vi "Add_Projection_Layer.vi"(4 "seed":i32=42, 6 "Proj_Dim":i32=256, 8 "error in (no error)":errorcluster, 11 "NN in":T1 {"LR_Update_Policy"."WarmUp_Ratio" min=1; "LR_Update_Policy"."WarmUp_Iter" min=1; "LR_Update_Policy"."LR0" format="%.7f"}) -> (0 "error out":errorcluster, 3 "NN out":T1 {"LR_Update_Policy"."WarmUp_Ratio" min=1; "LR_Update_Policy"."WarmUp_Iter" min=1; "LR_Update_Policy"."LR0" format="%.7f"})   [LabVIEW 2020]
uses:
  <vilib>/Ngene/Deep Learning Toolkit/Toolkit/NN_Network/Controls/NN.ctl
  <vilib>/Ngene/Deep Learning Toolkit/Toolkit/NN_Layers/Controls/NN_Layer_ref.ctl
  <vilib>/Ngene/Deep Learning Toolkit/Toolkit/NN_Layers/Controls/NN_Layer.ctl
  <vilib>/Ngene/Deep Learning Toolkit/Toolkit/NN_Layers/Controls/NN_Layer_Type.ctl
  <vilib>/Ngene/Deep Learning Toolkit/Toolkit/NN_Data/API/NN_Dims(C,H,W).ctl
  <vilib>/Ngene/Deep Learning Toolkit/Toolkit/NN_Layers/Controls/NN_Layer_Metrics.ctl
  <vilib>/Ngene/Deep Learning Toolkit/Toolkit/NN_Network/Controls/NN_Device.ctl
  <vilib>/Ngene/Deep Learning Toolkit/Toolkit/NNg/cuda/Controls/nng_cuda_handles.ctl
  <vilib>/Ngene/Deep Learning Toolkit/Toolkit/NN_Layers/Controls/NN_Layer_Dimty.ctl
  <vilib>/Ngene/Deep Learning Toolkit/Toolkit/NN_Layers/Controls/NN_Layer_RF_State.ctl
  <vilib>/Ngene/Deep Learning Toolkit/Toolkit/NN_Data/API/NN_Dims(V,H).ctl
  <vilib>/Ngene/Deep Learning Toolkit/Toolkit/NN_Network/Controls/NN_In_Out_Dim-ty.ctl
  <vilib>/Ngene/Deep Learning Toolkit/Toolkit/NN_Train/Controls/NN_Train_Params.ctl
  <vilib>/Ngene/Deep Learning Toolkit/Toolkit/NN_Train/Controls/NN_Train_Optimizer.ctl
  <vilib>/Ngene/Deep Learning Toolkit/Toolkit/NN_Train/Controls/NN_Train_Data_Sampling.ctl
  <vilib>/Ngene/Deep Learning Toolkit/Toolkit/NN_Train/Controls/NN_LR_Policy_Cfg.ctl
  <vilib>/Ngene/Deep Learning Toolkit/Toolkit/NN_Train/Controls/NN_LR_Policy_Type.ctl
  <vilib>/Ngene/Deep Learning Toolkit/Toolkit/NN_Train/Controls/NN_Train_Session_Data.ctl
  <vilib>/Ngene/Deep Learning Toolkit/Toolkit/NN_Data/Controls/NN_Ground_truth.ctl
  <vilib>/Ngene/Deep Learning Toolkit/Toolkit/NN_Train/Controls/NN_Loss_Type.ctl
  <vilib>/Ngene/Deep Learning Toolkit/Toolkit/NNg/Network/WS/Controls/NNG_WS.ctl
  <vilib>/Ngene/Deep Learning Toolkit/Toolkit/NNg/Network/WS/Controls/NNg_WS_Mem_DVR.ctl
  <vilib>/Ngene/Deep Learning Toolkit/Toolkit/NNg/cuda/Controls/cuda_Mem_desc.ctl
  <vilib>/Ngene/Deep Learning Toolkit/Toolkit/NN_Layers/Layers/Conv2D/Controls/NN_Layer_Config(Conv2D).ctl
  <vilib>/Ngene/Deep Learning Toolkit/Toolkit/NN_Layers/Layers/Conv2D/Controls/NN_Layer_Params(Conv2D).ctl
  <vilib>/Ngene/Deep Learning Toolkit/Toolkit/NN_Layers/Layers/Conv2D/Controls/NN_Conv2D_Padding_Type.ctl
  <vilib>/Ngene/Deep Learning Toolkit/Toolkit/NN_Layers/Layers/BatchNorm/Controls/NN_BN_Params.ctl
  <vilib>/Ngene/Deep Learning Toolkit/Toolkit/NN_Activations/Controls/NN_Activation_Type.ctl
  <vilib>/Ngene/Deep Learning Toolkit/Toolkit/NN_Layers/Controls/NN_Layer_Init_Params.ctl
  <vilib>/Ngene/Deep Learning Toolkit/Toolkit/NN_Layers/Controls/NN_Layer_Weight_Init_Type.ctl
  <vilib>/Ngene/Deep Learning Toolkit/Toolkit/NN_Layers/Layers/Conv2D/NN_Layer_Create(Conv2D).vi
  <vilib>/Ngene/Deep Learning Toolkit/Toolkit/NN_Layers/subVIs/Get_Weights/NN_Get_Weights(Conv2D).vi
  <vilib>/Ngene/Deep Learning Toolkit/Toolkit/NN_Data/subVIs/Get_Data_Vals/2D/NN_Data_Get_ValByRef(2D_SGL).vi
  <vilib>/Ngene/Deep Learning Toolkit/Toolkit/NN_Data/subVIs/Set_Data_Vals/2D/NN_Data_Set_ValByRef(2D_SGL).vi
  <vilib>/Ngene/Deep Learning Toolkit/Toolkit/Deep_Learning_Toolkit_by_Ngene.lvlib
  <vilib>/Analysis/NI_AALBase.lvlib
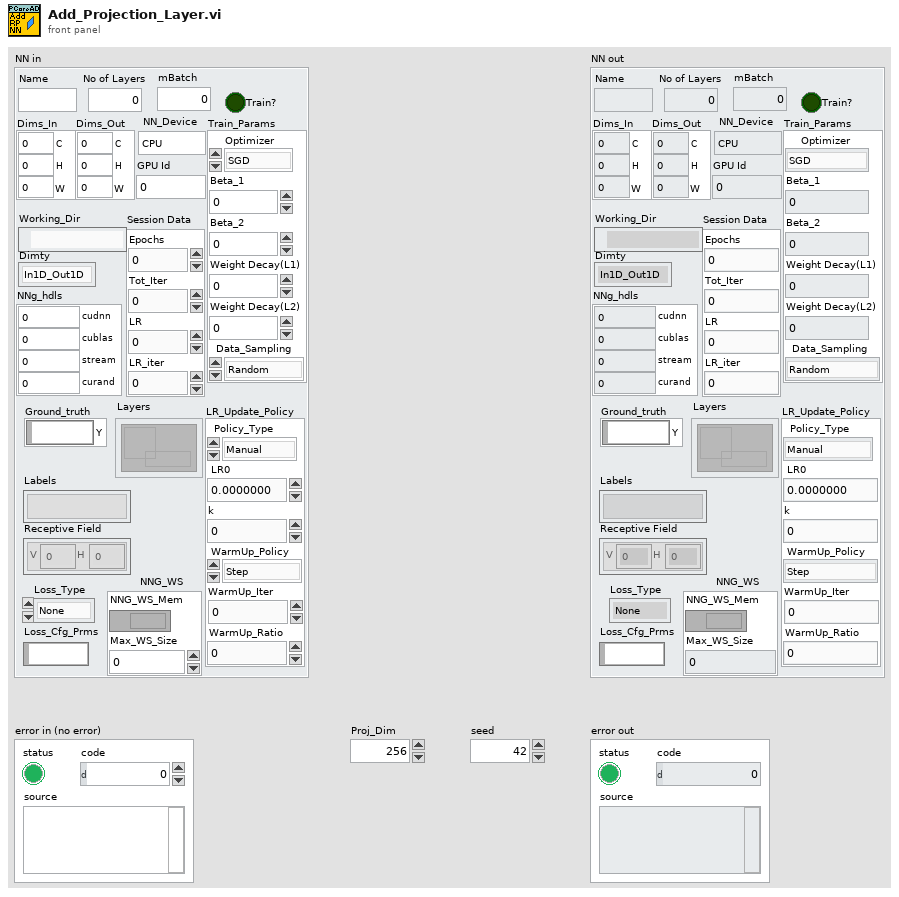
[diagram p1: front panel]
types:
  T1 = typedef "Deep_Learning_Toolkit_by_Ngene.lvlib/NN.ctl" = cluster{"Name":string, "No of Layers":i32, "mBatch":i32, "Layers":T2[], "Dimty":T3, "Dims_In":T4, "Dims_Out":T4, "Working_Dir":path, "Train?":bool, "Train_Params":T5, "LR_Update_Policy":T8, "Session Data":T10, "Ground_truth":T11, "NNg_hdls":T12, "NN_Device":T13, "GPU Id":i32, "Labels":string[], "Receptive Field":T14[], "Loss_Type":T15, "Loss_Cfg_Prms":variant, "NNG_WS":T16}
  T2 = typedef "Deep_Learning_Toolkit_by_Ngene.lvlib/NN_Layer_ref.ctl" = refnum<data-value>
  T3 = typedef "Deep_Learning_Toolkit_by_Ngene.lvlib/NN_In_Out_Dim-ty.ctl" = enum8{"In1D_Out1D", "In3D_Out1D", "In3D_Out3D", "In3D_OutBBox"}
  T4 = typedef "Deep_Learning_Toolkit_by_Ngene.lvlib/NN_Dims(C,H,W).ctl" = cluster{"C":i32, "H":i32, "W":i32}
  T5 = typedef "Deep_Learning_Toolkit_by_Ngene.lvlib/NN_Train_Params.ctl" = cluster{"Optimizer":T6, "Beta_1":sgl, "Beta_2":sgl, "Weight Decay(L1)":sgl, "Weight Decay(L2)":sgl, "Data_Sampling":T7}
  T6 = typedef "Deep_Learning_Toolkit_by_Ngene.lvlib/NN_Train_Optimizer.ctl" = enum16{"SGD", "Adam", "Adagrad", "Adadelta", "RMSProp", "Nesterov"}
  T7 = typedef "Deep_Learning_Toolkit_by_Ngene.lvlib/NN_Train_Data_Sampling.ctl" = enum16{"Random", "Sequential"}
  T8 = typedef "Deep_Learning_Toolkit_by_Ngene.lvlib/NN_LR_Policy_Cfg.ctl" = cluster{"Policy_Type":T9, "LR0":dbl, "k":sgl, "WarmUp_Policy":enum16{"Step", "Ramp"}, "WarmUp_Iter":i32, "WarmUp_Ratio":sgl}
  T9 = typedef "Deep_Learning_Toolkit_by_Ngene.lvlib/NN_LR_Policy_Type.ctl" = enum16{"Manual", "Step", "Exp", "1/t"}
  T10 = typedef "Deep_Learning_Toolkit_by_Ngene.lvlib/NN_Train_Session_Data.ctl" = cluster{"Epochs":sgl, "Tot_Iter":i32, "LR":sgl, "LR_iter":i32}
  T11 = typedef "Deep_Learning_Toolkit_by_Ngene.lvlib/NN_Ground_truth.ctl" = cluster{"Y":variant}
  T12 = typedef "Deep_Learning_Toolkit_by_Ngene.lvlib/nng_cuda_handles.ctl" = cluster{"cudnn":u64, "cublas":u64, "stream":u64, "curand":u64}
  T13 = typedef "Deep_Learning_Toolkit_by_Ngene.lvlib/NN_Device.ctl" = enum16{"CPU", "GPU"}
  T14 = typedef "Deep_Learning_Toolkit_by_Ngene.lvlib/NN_Dims(V,H).ctl" = cluster{"V":i32, "H":i32}
  T15 = typedef "Deep_Learning_Toolkit_by_Ngene.lvlib/NN_Loss_Type.ctl" = enum16{"None", "MSE", "CrossEntropy", "YOLO_v2", "YOLO_v4"}
  T16 = typedef "Deep_Learning_Toolkit_by_Ngene.lvlib/NNG_WS.ctl" = cluster{"NNG_WS_Mem":T17, "Max_WS_Size":i64}
  T17 = typedef "Deep_Learning_Toolkit_by_Ngene.lvlib/NNg_WS_Mem_DVR.ctl" = refnum<data-value>
  T18 = typedef "Deep_Learning_Toolkit_by_Ngene.lvlib/NN_Layer_Config(Conv2D).ctl" = cluster{"Name":string, "Conv_Params":T19, "BN?":bool, "BN_Params":T21, "Activation":T22, "Has Bias?":bool, "Init_Params":T23, "Custom_Params":string}
  T19 = typedef "Deep_Learning_Toolkit_by_Ngene.lvlib/NN_Layer_Params(Conv2D).ctl" = cluster{"Filters":i32, "Kernel_Size":i32, "Stride":i32, "Pad_Type":T20, "Pad_Size":i32}
  T20 = typedef "Deep_Learning_Toolkit_by_Ngene.lvlib/NN_Conv2D_Padding_Type.ctl" = enum16{"Pad_Size", "Valid", "Same"}
  T21 = typedef "Deep_Learning_Toolkit_by_Ngene.lvlib/NN_BN_Params.ctl" = cluster{"epsilon":sgl, "momentum":sgl}
  T22 = typedef "Deep_Learning_Toolkit_by_Ngene.lvlib/NN_Activation_Type.ctl" = enum16{"Sigmoid", "ReLU", "LReLU", "ReLU6", "tanh", "Swish", "Mish", "None"}
  T23 = typedef "Deep_Learning_Toolkit_by_Ngene.lvlib/NN_Layer_Init_Params.ctl" = cluster{"Init_Type":T24, "Value":sgl}
  T24 = typedef "Deep_Learning_Toolkit_by_Ngene.lvlib/NN_Layer_Weight_Init_Type.ctl" = enum16{"Const", "Uniform", "Gaussian", "Xavier"}
  T25 = typedef "Deep_Learning_Toolkit_by_Ngene.lvlib/NN_Layer.ctl" = cluster{"Name":string, "Layer_Data":variant, "Layer_Type":T26, "Dims_In":T4, "Layers_In":variant, "Dims_Out":T4, "Layers_Out":variant, "Metrics":T27, "GPU_Data":variant, "mBatch":i32, "NN_Device":T13, "NNg_hdls":T12, "Train?":bool, "Dimty":T28, "RecptField":T29}
  T26 = typedef "Deep_Learning_Toolkit_by_Ngene.lvlib/NN_Layer_Type.ctl" = enum16{"Input1D", "Input3D", "Conv1D", "Conv2D", "Conv2D_Adv", "MaxPool", "AvgPool", "UpSample", "DropOut3D", "ShortCut", "Concat", "SoftMax3D", "FC", "DropOut", "Softmax", "Flatten", "YOLO_v2", "YOLO_v4", "Activation", "BatchNormalization", "Unsupported"}
  T27 = typedef "Deep_Learning_Toolkit_by_Ngene.lvlib/NN_Layer_Metrics.ctl" = cluster{"Data":dbl, "Params":dbl, "Ops":dbl}
  T28 = typedef "Deep_Learning_Toolkit_by_Ngene.lvlib/NN_Layer_Dimty.ctl" = enum16{"1D", "3D"}
  T29 = typedef "Deep_Learning_Toolkit_by_Ngene.lvlib/NN_Layer_RF_State.ctl" = cluster{"Dims":T14, "J":T14}
  T30 = typedef "Deep_Learning_Toolkit_by_Ngene.lvlib/NN_Layer_Weights(ref).ctl" = cluster{"W":T31, "b":T32, "BN_ref":T33}
  T31 = typedef "Deep_Learning_Toolkit_by_Ngene.lvlib/NN_Data_ref(2D_SGL).ctl" = refnum<data-value>
  T32 = typedef "Deep_Learning_Toolkit_by_Ngene.lvlib/NN_Data_ref(1D_SGL).ctl" = refnum<data-value>
  T33 = typedef "Deep_Learning_Toolkit_by_Ngene.lvlib/NN_BN(ref).ctl" = cluster{"scales(ref)":T32, "roll_mean(ref)":T32, "roll_var(ref)":T32, "bias(ref)":T32}
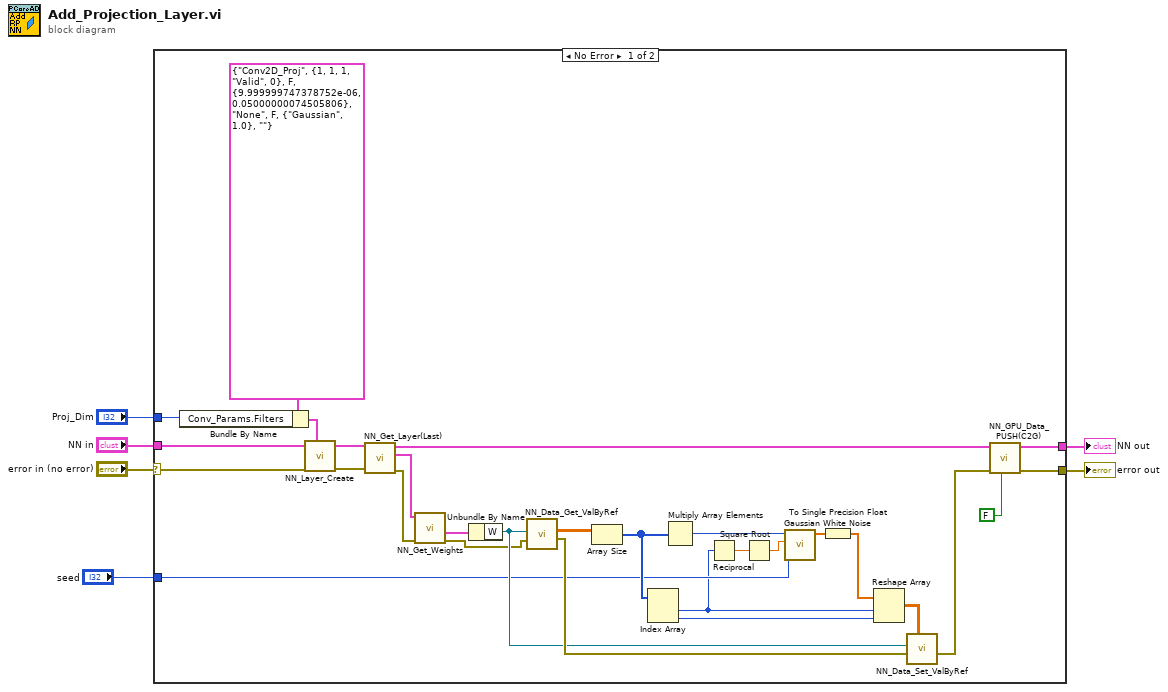
[diagram p0: block diagram]
diagram:
  n1 = case shown="No Error" "error in (no error)" {
    selector: "error in (no error)" -> [w16 w37]
    tunnel: [w7 w37] -> w6
    tunnel: [w9 w36] -> w5
    tunnel: "NN in" -> [w25 w36]
    tunnel: "Proj_Dim" -> [w17 _]
    tunnel: "seed" -> [w15 _]
    frame No Error {
      n2 = Bundle By Name(cluster=T18 {"Name"="Conv2D_Proj", "Conv_Params"={"Filters"=1, "Kernel_Size"=1, "Stride"=1, "Pad_Type"=enum."Valid", "Pad_Size"=0}, "BN?"=FALSE, "BN_Params"={"epsilon"=1e-05, "momentum"=0.05}, "Activation"=enum."None", "Has Bias?"=FALSE, "Init_Params"={"Init_Type"=enum."Gaussian", "Value"=1.0}, "Custom_Params"=""} ("Conv2D_Cfg"), "Conv_Params.Filters"=w17) -> (w22:T18)
      n3 = call-poly <vilib>:"NN_Layer_Create.vi"("Conv2D_Cfg"=w22, "error in (no error)"=w16, "NN in"=w25) -> ("error out"=w33:errorcluster, "NN out"=w19:T1)  [unwired: 6 in, 1 out]
      n4 = call <vilib>:"NN_Get_Layer(Last).vi"("error in (no error)"=w33, "NN in"=w19) -> ("error out"=w34:errorcluster, "Last_Layer"=w20:T25, "NN out"=w10:T1)  [unwired: 6 in, 1 out]
      n5 = call-poly <vilib>:"NN_Get_Weights.vi"("error in (no error)"=w34, "Layer(Conv2D)"=w20) -> ("error out"=w13:errorcluster, "Weights_refs"=w21:T30)  [unwired: 7 in, 1 out]
      n6 = Unbundle By Name(w21) -> ("W"=w23:T31)
      n7 = call-poly <vilib>:"NN_Data_Get_ValByRef.vi"("error in (no error)"=w13, "DVR(2D_SGL)"=w23) -> ("error out"=w35:errorcluster, "Value(2D_SGL)"=w24:sgl[][])  [unwired: 6 in]
      n8 = Array Size(array=w24) -> (size(s)=w27:i32[])
      n9 = Index Array(array=w27) -> (element #1=w14:i32, element #2=w12:i32)  [unwired: 2 in]
      n10 = Multiply Array Elements(1:w27) -> (0:w26:i32)
      n11 = Reciprocal(x=w14) -> (1/x=w28:dbl)
      n12 = Square Root(x=w28) -> (sqrt(x)=w29:dbl)
      n13 = call <vilib>:"Gaussian White Noise.vi"("seed"=w15, "standard deviation"=w29, "samples"=w26) -> ("Gaussian noise pattern"=w30:dbl[])  [unwired: 7 in, 1 out]
      n14 = To Single Precision Float(number=w30) -> (single precision float=w32:sgl[])
      n15 = Reshape Array(w32, w14, w12) -> (w31:sgl[][])
      n16 = call-poly <vilib>:"NN_Data_Set_ValByRef.vi"("Value(2D_SGL)"=w31, "error in (no error)"=w35, "DVR(2D_SGL)"=w23) -> ("error out"=w8:errorcluster)  [unwired: 8 in]
      n17 = call <vilib>:"NN_GPU_Data_PUSH(C2G).vi"("All Data?"=FALSE, "error in (no error)"=w8, "NN in"=w10) -> ("error out"=w7:errorcluster, "NN out"=w9:T1)  [unwired: 7 in]
    }
    frame Error {
    }
  }
  "error out" <- w6
  "NN out" <- w5
